vi "SaveExpConfig.vi"(8 "error in (no error)":errorcluster caption="entrée d'erreur", 9 "Experiment":path, 11 "Experiment.lvclass":refnum<class "Experiment.lvclass">) -> (0 "error out":errorcluster caption="sortie d'erreur", 3 "Experiment.lvclass 2":refnum<class "Experiment.lvclass">)   [LabVIEW 2019, in "Experiment.lvclass"]
uses:
  Experiment.lvclass
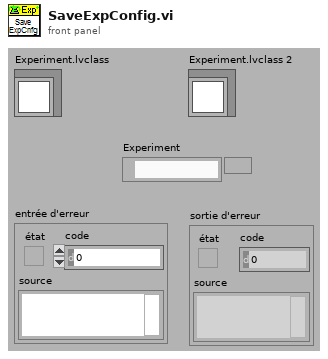
[diagram p1: front panel]
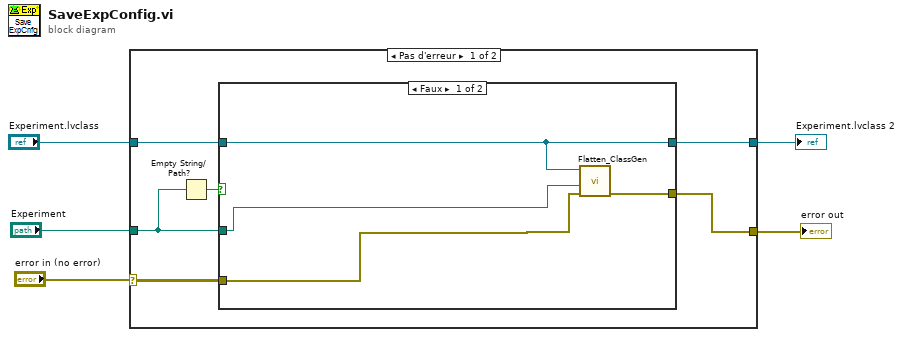
[diagram p0: block diagram]
diagram:
  n1 = case shown="Pas d'erreur" "error in (no error)" {
    selector: "error in (no error)" -> [w8 w19]
    tunnel: "Experiment.lvclass" -> [w10 w18]
    tunnel: [w11 w19] -> w5
    tunnel: [w9 w18] -> w2
    tunnel: "Experiment" -> [w6 _]
    frame No Error {
      n2 = Empty String/Path?(string/path=w6) -> (empty?=w7:bool)
      n3 = case shown="Faux" w7 {
        tunnel: [w15 w16] -> w11
        tunnel: w10 -> [w14 w17]
        tunnel: [w14 w17] -> w9
        tunnel: w8 -> [w12 w16]
        tunnel: w6 -> [w13 _]
        frame False {
          n4 = call <userlib>:"Flatten_ClassGen.vi"("error in (no error)"=w12, "XML File Path"=w13, "Objet LabVIEW"=w14) -> ("error out"=w15:errorcluster)  [unwired: 6 in, 2 out]
        }
        frame True {
        }
      }
    }
    frame Error {
    }
  }
  "error out" <- w5
  "Experiment.lvclass 2" <- w2
